vi "BRPopLPush.vi"(0 "reference in":refnum<class "Redis.lvclass">, 5 "Source":string, 9 "Destination":string, 11 "Error In":errorcluster, 13 "Timeout(1000ms)":i32=1000) -> (4 "reference out":refnum<class "Redis.lvclass">, 8 "Return":string, 15 "Error Out":errorcluster)   [LabVIEW 2020, in "Redis.lvclass"]
doc: "<b>BRPOPLPUSH</b>\n\nBRPOPLPUSH is the blocking variant of RPOPLPUSH. When source contains elements, this command behaves exactly like RPOPLPUSH. When used inside a MULTI/EXEC block, this command behaves exactly like RPOPLPUSH. When source is empty, Redis will block the connection until another client pushes to it or until timeout is reached. A timeout of zero can be used to block indefinitely.\n\nSee RPOPLPUSH for more information."
uses:
  Redis.lvclass
  Redis.lvclass/Redis.ctl
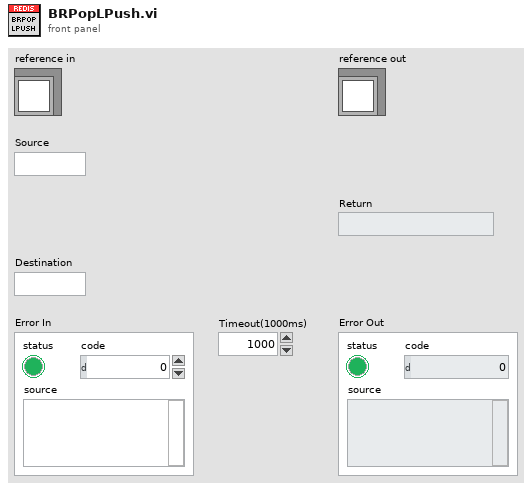
[diagram p1: front panel]
types:
  T1 = typedef "Redis.lvclass/RedisDataType.ctl" = cluster{"Reply Type":T2, "Integer":i64, "String":string, "Multibulk":variant[], "StringData":string[]}
  T2 = typedef "Redis.lvclass/ReplyDataTypeEnum.ctl" = enum16{"None", "Error", "Status", "Nil", "Integer", "String", "Multibulk"}
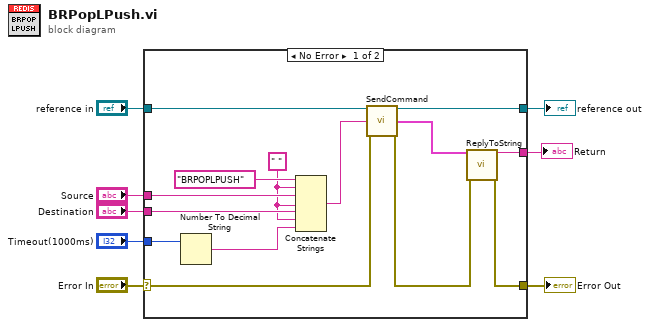
[diagram p0: block diagram]
diagram:
  n1 = case shown="No Error" "Error In" {
    selector: "Error In" -> [w20 w24]
    tunnel: [w12 w24] -> w7
    tunnel: [w22 w23] -> w5
    tunnel: "reference in" -> [w21 w23]
    tunnel: "Source" -> [w18 _]
    tunnel: "Destination" -> [w16 _]
    tunnel: [w14 _] -> w2
    tunnel: "Timeout(1000ms)" -> [w10 _]
    frame No Error {
      w11 = " "
      n2 = Number To Decimal String(number=w10) -> (decimal integer string=w9:string)  [unwired: 1 in]
      n3 = Concatenate Strings("BRPOPLPUSH", w11, w18, w11, w16, w11, w9) -> (w17:string)
      n4 = call "SendCommand.vi"("reference in"=w21, "Command"=w17, "Error In"=w20) -> ("reference out"=w22:refnum<class "Redis.lvclass">, "Data"=w15:T1, "Error Out"=w13:errorcluster)  [unwired: 10 in]
      n5 = call "ReplyToString.vi"("Reply"=w15, "Error In"=w13) -> ("String"=w14:string, "Error Out"=w12:errorcluster)  [unwired: 12 in]
    }
    frame Error {
    }
  }
  "Error Out" <- w7
  "reference out" <- w5
  "Return" <- w2
